vi "KDC101_GetStatus.vi"(8 "error in (no error)":errorcluster caption="entrée d'erreur (pas d'erreur)", 11 "KCubeDCServoRef":refnum<k24>) -> (0 "error out":errorcluster caption="sortie d'erreur", 1 "Homed":bool, 2 "ActPos(Deg)":dbl=60.0 caption="ActPos(deg)" min=0.1 step=0.1 format="%#.1f", 3 "KCubeDCServoRefOut":refnum<k24>, 4 "Moving":bool)   [LabVIEW 2019]
doc: "Utilisez ce modèle pour construire un VI à utiliser en tant que sous-VI."
uses:
  C:/Program Files (x86)/National Instruments/LabVIEW 2019/user.lib/ThorKDC101/Kinesis_with_LabVIEW_Examples_LV12 - v3/ThorLabs.MotionControl.KCube.DCServoCLI.dll
  Kinesis_with_LabVIEW_Examples_LV12 - v3/ThorLabs.MotionControl.KCube.DCServoCLI.dll
  C:/Program Files (x86)/National Instruments/LabVIEW 2019/user.lib/ThorKDC101/Kinesis_with_LabVIEW_Examples_LV12 - v3/Thorlabs.MotionControl.GenericMotorCLI.dll
  Kinesis_with_LabVIEW_Examples_LV12 - v3/Thorlabs.MotionControl.GenericMotorCLI.dll
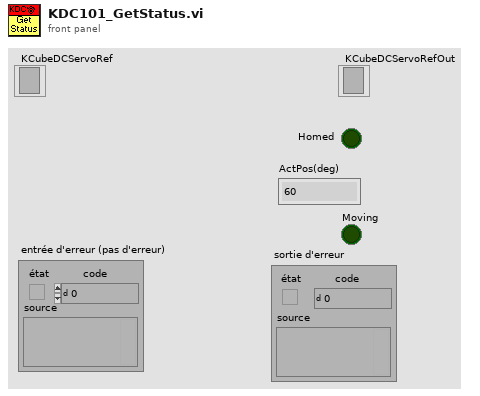
[diagram p1: front panel]
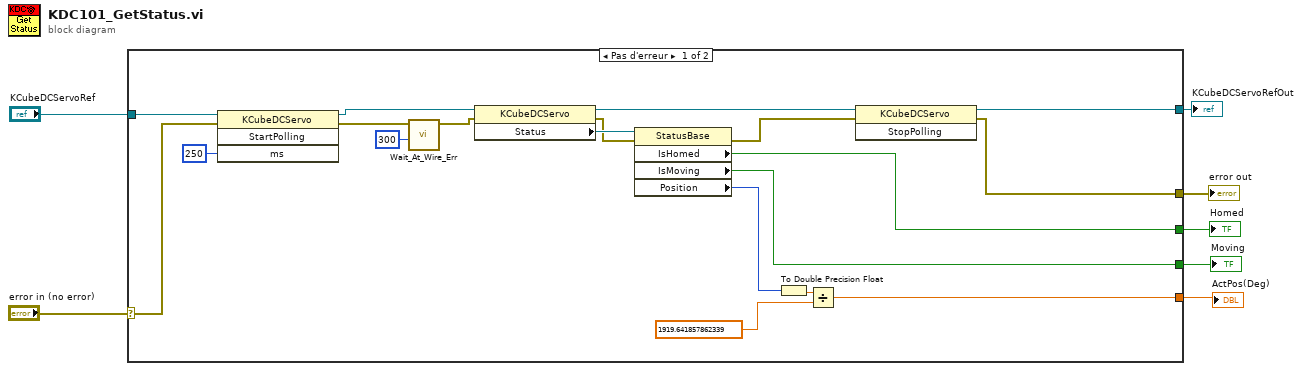
[diagram p0: block diagram]
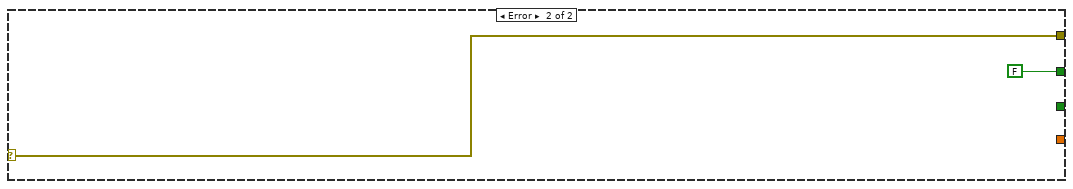
[diagram p2: hidden frame]
diagram:
  n1 = case shown="Pas d'erreur" "error in (no error)" {
    selector: "error in (no error)" -> [w15 w28]
    tunnel: [w9 w28] -> w6
    tunnel: [w21 FALSE] -> w5
    tunnel: "KCubeDCServoRef" -> [w16 _]
    tunnel: [w18 _] -> w3
    tunnel: [w17 _] -> w2
    tunnel: [w8 _] -> w1
    frame No Error {
      n2 = invoke class="KCubeDCServo" method="StartPolling"(reference=w16, error in=w15, "ms"=250) -> (reference out=w22:refnum<k24>, error out=w23:errorcluster)  [unwired: 1 in, 2 out]
      n3 = call <userlib>:"Wait_At_Wire_Err.vi"("Wait (ms)"=u32 300, "error in (no error)"=w23) -> ("error out"=w25:errorcluster)  [unwired: 7 in, 2 out]
      n4 = property class="KCubeDCServo"(reference=w22, error in=w25) -> (reference out=w19:refnum<k24>, error out=w13:errorcluster, "Status"=w14:refnum<k24>)
      n5 = property class="StatusBase"(reference=w14, error in=w13) -> (error out=w20:errorcluster, "IsHomed"=w21:bool, "IsMoving"=w8:bool, "Position"=w11:i64)  [unwired: 1 out]
      n6 = To Double Precision Float(number=w11) -> (double precision float=w12:dbl)
      n7 = Divide(x=w12, y=1919.641857862339) -> (x/y=w17:dbl)
      n8 = invoke class="KCubeDCServo" method="StopPolling"(reference=w19, error in=w20) -> (reference out=w18:refnum<k24>, error out=w9:errorcluster)  [unwired: 1 in, 1 out]
    }
    frame Error {
    }
  }
  "error out" <- w6
  "Homed" <- w5
  "KCubeDCServoRefOut" <- w3
  "ActPos(Deg)" <- w2
  "Moving" <- w1
